vi "Teleop.vi"(10 "Match Info":T1={"Autonomous Elapsed Seconds"=0.0, "TeleOp Elapsed Seconds"=0.0, "Disabled Elapsed Seconds"=0.0, "Visited Autonomous"=FALSE, "Visited TeleOp"=FALSE, "Visited Disabled"=FALSE, "Autonomous Settings"={"Autonomous Style"=enum."Independent", "VI Refnum"=refnum}}, 11 "Call Context":T2) -> ()   [LabVIEW 2013]
doc: "This VI is called for each TeleOp packet received from the DS where the robot is not disabled. It is often used to read from the joysticks and update I/O or to update setpoints for timed control loops. It should complete and return within 20 milliseconds or it may miss DS packets."
uses:
  <vilib>/Rock Robotics/WPI/DriverStation/WPI_DriverStationDerivedRobotMode.ctl
  <vilib>/Rock Robotics/WPI/DriverStation/WPI_DriverStationMatch Info.ctl
  871/Utils/GetSetType.ctl
  <vilib>/Rock Robotics/WPI/Relay/WPI_RelayValue.ctl
  Robot Global Data.vi
  <vilib>/Rock Robotics/WPI/RobotDrive/WPI_RobotDriveMecanumDrive_Polar.vi
  <vilib>/Rock Robotics/WPI/Joystick/WPI_JoystickGetSetRefNum.vi
  <vilib>/Rock Robotics/WPI/RobotDrive/WPI_RobotDriveGetSetRefNum.vi
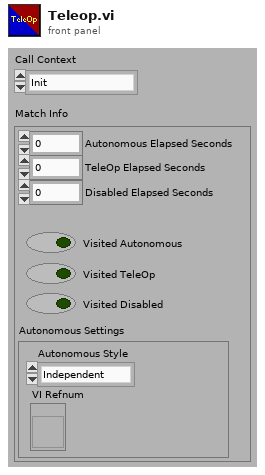
[diagram p1: front panel]
types:
  T1 = typedef "WPI_DriverStationMatch Info.ctl" = cluster{"Autonomous Elapsed Seconds":dbl, "TeleOp Elapsed Seconds":dbl, "Disabled Elapsed Seconds":dbl, "Visited Autonomous":bool, "Visited TeleOp":bool, "Visited Disabled":bool, "Autonomous Settings":cluster{"Autonomous Style":enum16{"Iterative", "Independent"}, "VI Refnum":refnum<vi>}}
  T2 = typedef "WPI_DriverStationDerivedRobotMode.ctl" = enum16{"Init", "Execute", "Stop"}
  T3 = typedef "WPI_RelayValue.ctl" = enum16{"Off", "On", "Forward", "Reverse"}
  T4 = typedef "GetSetType.ctl" = enum16{"Get", "Set"}
  T5 = typedef "WPI_JoystickDevRef.ctl" = cluster{"Device":T6}
  T6 = typedef "WPI_JoystickDeviceEnum.ctl" = enum16{"USB 1", "USB 2", "USB 3", "USB 4", "Kinect 1", "Kinect 2"}
  T7 = typedef "XBox Buttons.ctl" = cluster{"Y":bool, "B":bool, "A":bool, "X":bool, "RB":bool, "LB":bool, "START":bool, "SELECT":bool, "R3":bool, "L3":bool}
  T8 = typedef "Xbox Axis.ctl" = cluster{"Left Stick X":dbl, "Left Stick Y":dbl, "Right stick X":dbl, "Right Stick Y":dbl, "Trigger":dbl}
  T9 = typedef "WPI_DigitalInputDevRef.ctl" = cluster{"DevStatus":errorcluster, "DIO Channel":T10, "Digital Module":T11}
  T10 = typedef "FPGA_DIOChannel.ctl" = enum8{"DIO 1", "DIO 2", "DIO 3", "DIO 4", "DIO 5", "DIO 6", "DIO 7", "DIO 8", "DIO 9", "DIO 10", "DIO 11", "DIO 12", "DIO 13", "DIO 14", "Invalid"}
  T11 = typedef "FPGA_TypedefDigitalModule.ctl" = enum16{"Digital Module 1", "Digital Module 2"}
  T12 = typedef "WPI_MotorControlDeviceRef.ctl" = cluster{"DeviceStatus":errorcluster, "Type":enum16{"PWM", "CAN"}, "PWM":cluster{"Digital Module":T11, "PWM Channel":T13, "DeadBand":T14}, "CAN":cluster{"Device Number":u8, "Control Mode":T15, "Semaphore":T16, "Max Vout":dbl}, "Invert":bool, "TransformRef":T17, "InvTransformRef":T17}
  T13 = typedef "FPGA_DIOPWMChannel.ctl" = enum8{"PWM 1", "PWM 2", "PWM 3", "PWM 4", "PWM 5", "PWM 6", "PWM 7", "PWM 8", "PWM 9", "PWM 10", "Invalid"}
  T14 = typedef "WPI_PWMDeadband.ctl" = cluster{"Name":string, "maxPositivePwm":i32, "minPositivePwm":i32, "centerPwm":i32, "maxNegativePwm":i32, "minNegativePwm":i32, "angularRange":u16}
  T15 = typedef "WPI_CANJaguar_ControlMode.ctl" = enum8{"Percent VBus", "Current", "Speed", "Position", "Voltage"}
  T16 = typedef "Semaphore RefNum" = refnum<k1>
  T17 = typedef "WPI_PWMTransform_ConPane.ctl" = refnum<vi>
  T18 = typedef "WPI_GyroDevRef.ctl" = cluster{"DevStatus":errorcluster, "Analog Module":T19, "Analog Channel":T20, "Offset":dbl, "Gain (VoltsPerDegree/Second)":dbl}
  T19 = typedef "FPGA_TypedefAnalogModule.ctl" = enum16{"Analog Module 1", "Analog Module 2"}
  T20 = typedef "FPGA_AIChannel.ctl" = enum8{"AI 1", "AI 2", "AI 3", "AI 4", "AI 5", "AI 6", "AI 7", "AI 8", "Invalid"}
  T21 = typedef "Targetsss.ctl" = cluster{"Vertical Target":T22, "Horizontal Target":T22, "Valid?":bool, "Scores":T23, "Hot?":bool}
  T22 = typedef "Target Type.ctl" = cluster{"Area":dbl, "Bounding box":cluster{"BB Left":dbl, "BB Top":dbl, "BB Right":dbl, "BB Bottom":dbl}, "Center of Mass":cluster{"X Value":dbl, "Y Value":dbl}, "Equivilent Rectangle":cluster{"Width":dbl, "Height":dbl}, "Aspect Ratio":dbl, "Rectangularity":dbl, "Horizontal?":bool}
  T23 = typedef "Scores.ctl" = cluster{"Score Total":dbl, "Left Score":dbl, "Right Score":dbl, "Vertical Score":dbl, "Index":dbl}
  T24 = typedef "WPI_RelayDevRef.ctl" = cluster{"DevStatus":errorcluster, "Relay Channel":T25, "Digital Module":T11, "Relay Direction":T26}
  T25 = typedef "FPGA_DIORelayChannel.ctl" = enum8{"Relay 1", "Relay 2", "Relay 3", "Relay 4", "Relay 5", "Relay 6", "Relay 7", "Relay 8", "Invalid"}
  T26 = typedef "WPI_RelayDirection.ctl" = enum16{"Both directions", "Forward only", "Reverse only"}
  T27 = typedef "WPI_RobotDriveDevRef.ctl" = cluster{"DevStatus":errorcluster, "Motors[]":T12[], "Square Inputs":bool, "Max Output":dbl, "Isochronous":bool}
  T28 = typedef "ShooterDevRef.ctl" = cluster{"Wench Motor":T12, "Lower Wench Limit":T9, "Clutch Engaged Sensor":T9, "Worm Motor":T12, "Worm Screw Out Sensor":T9, "Clutch Disengaged Sensor":T9}
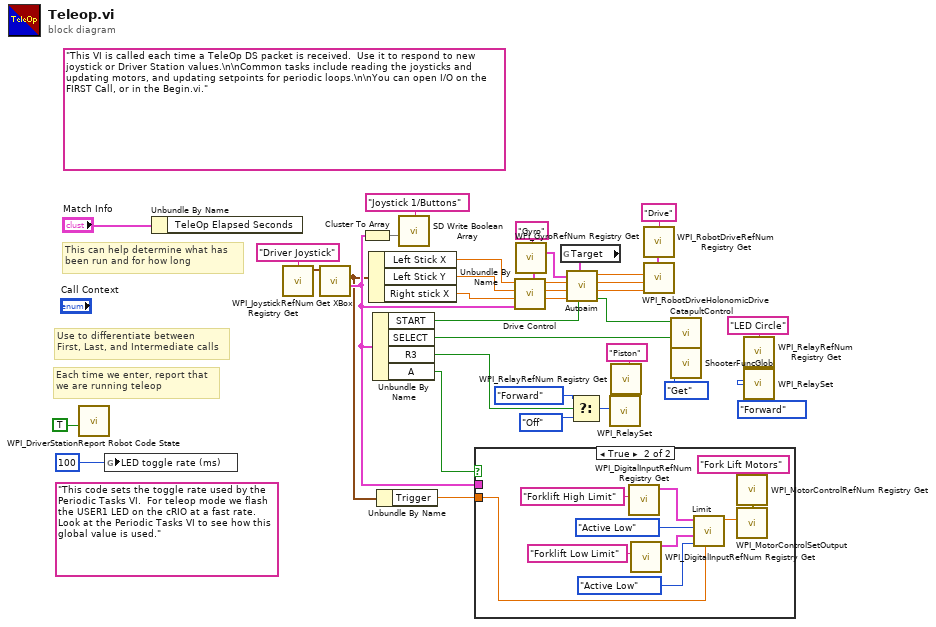
[diagram p0: block diagram]
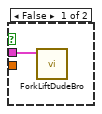
[diagram p2: hidden frame]
diagram:
  (unwired) "This code sets the toggle rate used by the Periodic Tasks VI.  For teleop mode we flash the USER1 LED on the cRIO at a fast rate.  Look at the Periodic Tasks VI to see how this global value is used."
  (unwired) "This VI is called each time a TeleOp DS packet is received.  Use it to respond to new joystick or Driver Station values.\n\nCommon tasks include reading the joysticks and updating motors, and updating setpoints for periodic loops.\n\nYou can open I/O on the FIRST Call, or in the Begin.vi."
  # "Each time we enter, report that\nwe are running teleop"
  # "Use to differentiate between\nFirst, Last, and Intermediate calls"
  # "This can help determine what has\nbeen run and for how long"
  n1 = call <vilib>:"WPI_DriverStationReport Robot Code State.vi"("TeleOp"=TRUE ("Autonomous")) -> ()  [unwired: 10 in, 1 out]
  n2 = global write "Robot Global Data.vi" "LED toggle rate (ms)"(u32 100 ("LED ms toggle rate")) -> ()
  n3 = Unbundle By Name("Match Info") -> ()  [unwired: 1 out]
  n4 = call <vilib>:"WPI_JoystickRefNum Registry Get.vi"("refnum name"="Driver Joystick") -> ("JoystickDevRef"=w35:T5)  [unwired: 1 in, 9 out]
  n5 = call "Get XBox.vi"("JoystickDevRefIn"=w35) -> ("Buttons"=w17:T7, "Axes"=w14:T8)  [unwired: 8 in, 1 out]
  n6 = Cluster To Array(cluster=w17) -> (array=w16:bool[])
  n7 = Unbundle By Name(w14) -> ("Left Stick X"=w33:dbl, "Left Stick Y"=w34:dbl, "Right stick X"=w32:dbl)
  n8 = Unbundle By Name(w17) -> ("START"=w9:bool, "SELECT"=w15:bool, "R3"=w1:bool, "A"=w2:bool)
  n9 = Unbundle By Name(w14) -> ("Trigger"=w13:dbl)
  n10 = call <vilib>:"SD Write Boolean Array.vi"("Boolean Array"=w16, "Name"="Joystick 1/Buttons") -> ()  [unwired: 8 in, 2 out]
  n11 = case shown="True" w2 {
    tunnel: w17 -> [w42 _]
    tunnel: w13 -> [_ w44]
    frame False {
      n12 = call "ForkLiftDudeBro.vi"("Buttons"=w42) -> ()  [unwired: 11 in]
    }
    frame True {
      n13 = call <vilib>:"WPI_DigitalInputRefNum Registry Get.vi"("refnum name"="Forklift High Limit") -> ("DigitalInputDevRef"=w48:T9)  [unwired: 9 in, 1 out]
      n14 = call <vilib>:"WPI_DigitalInputRefNum Registry Get.vi"("refnum name"="Forklift Low Limit") -> ("DigitalInputDevRef"=w45:T9)  [unwired: 9 in, 1 out]
      n15 = call "Limit.vi"("Input"=w44, "Lower sensor sense"=enum16{"Active Low", "Active High"}."Active Low", "Lower DigitalInputDevRef"=w45, "Upper sensor sense"=enum16{"Active Low", "Active High"}."Active Low", "Upper DigitalInputDevRef"=w48) -> ("Output"=w43:dbl)  [unwired: 6 in]
      n16 = call <vilib>:"WPI_MotorControlRefNum Registry Get.vi"("refnum name"="Fork Lift Motors") -> ("error out"=w52:errorcluster, "MotorControlDevRef"=w51:T12)  [unwired: 9 in]
      n17 = call <vilib>:"WPI_MotorControlSetOutput.vi"("error in (no error)"=w52, "Output"=w43, "MotorControlDevRef"=w51) -> ()  [unwired: 6 in, 3 out]
    }
  }
  n18 = call <vilib>:"WPI_GyroRefNum Registry Get.vi"("refnum name"="Gyro") -> ("GyroDevRef"=w12:T18)  [unwired: 9 in, 1 out]
  n19 = call "Drive Control.vi"("GyroDevRef"=w12, "Buttons"=w17, "rotation"=w32, "y"=w34, "x"=w33) -> ("Rotation"=w11:dbl, "Direction"=w27:dbl, "Speed"=w28:dbl)  [unwired: 4 in]
  n20 = global read "Robot Global Data.vi" "Target"() -> (w29:T21)
  n21 = call "Autoaim.vi"("Autoaim"=w9, "GyroDevRef"=w12, "Rotation"=w11, "Driver Direction"=w27, "Driver Magnitude"=w28, "Targetssssss"=w29) -> ("Are We There Yet?"=w23:bool, "Rotation"=w10:dbl, "Direction"=w25:dbl, "Magnitude"=w26:dbl)  [unwired: 2 in]
  n22 = Select(t=WPI_RelayValue."Forward" ("RelayValue"), s=w1, f=WPI_RelayValue."Off" ("RelayValue")) -> (s? t:f=w5:T3)
  n23 = call <vilib>:"WPI_RelayRefNum Registry Get.vi"("refnum name"="Piston") -> ("error out"=w8:errorcluster, "RelayDevRef"=w7:T24)  [unwired: 9 in]
  n24 = call <vilib>:"WPI_RelaySet.vi"("error in (no error)"=w8, "RelayValue"=w5, "RelayDevRef"=w7) -> ()  [unwired: 7 in, 2 out]
  n25 = call <vilib>:"WPI_RobotDriveRefNum Registry Get.vi"("refnum name"="Drive") -> ("RobotDriveDevRef"=w39:T27)  [unwired: 1 in, 9 out]
  n26 = call-poly <vilib>:"WPI_RobotDriveHolonomicDrive.vi"("Rotation"=w10, "Direction"=w25, "Magnitude"=w26, "RobotDriveDevRef"=w39) -> ()  [unwired: 5 in, 3 out]
  n27 = call "ShooterFuncGlob.vi"("Operation"=GetSetType."Get") -> ("ShooterDevRefOut"=w24:T28)  [unwired: 10 in]
  n28 = call "CatapultControl.vi"("Fire Button"=w15, "ShooterDevRefIn"=w24, "Are we there yet?"=w23) -> ()  [unwired: 9 in]
  n29 = call <vilib>:"WPI_RelayRefNum Registry Get.vi"("refnum name"="LED Circle") -> ("error out"=w20:errorcluster, "RelayDevRef"=w21:T24)  [unwired: 9 in]
  n30 = call <vilib>:"WPI_RelaySet.vi"("error in (no error)"=w20, "RelayValue"=WPI_RelayValue."Forward", "RelayDevRef"=w21) -> ()  [unwired: 7 in, 2 out]
